vi "BuildConstructor.vi"(7 "PythonConverter_BD in":refnum<class "PyConvBD.lvclass">, 8 "error in":errorcluster, 11 "Function in":refnum<class "GrowableFunction.lvclass">) -> (0 "error out":errorcluster, 3 "Function out":refnum<class "GrowableFunction.lvclass">, 4 "constructor":string, 5 "PythonConverter_BD out":refnum<class "PyConvBD.lvclass">)   [LabVIEW 2014, in "GrowableFunction.lvclass"]
uses:
  GrowableFunction.lvclass
  Python/PythonConverter_BD/PyConvBD.lvclass
  Python/Parsing/Classes/PythonFunction/PythonFunction.lvclass/PythonFunction.ctl
  Python/Parsing/Classes/PythonFunction/PythonFunction.lvclass
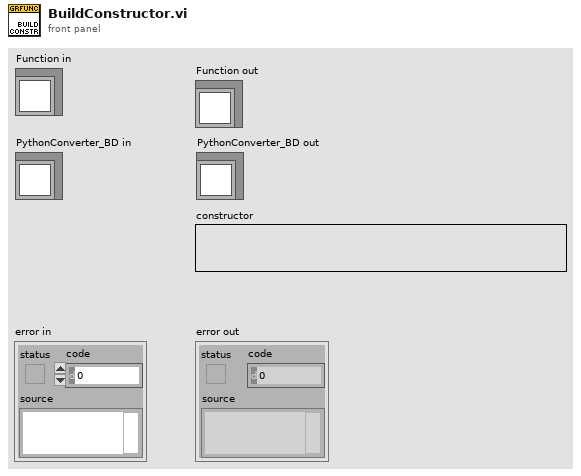
[diagram p1: front panel]
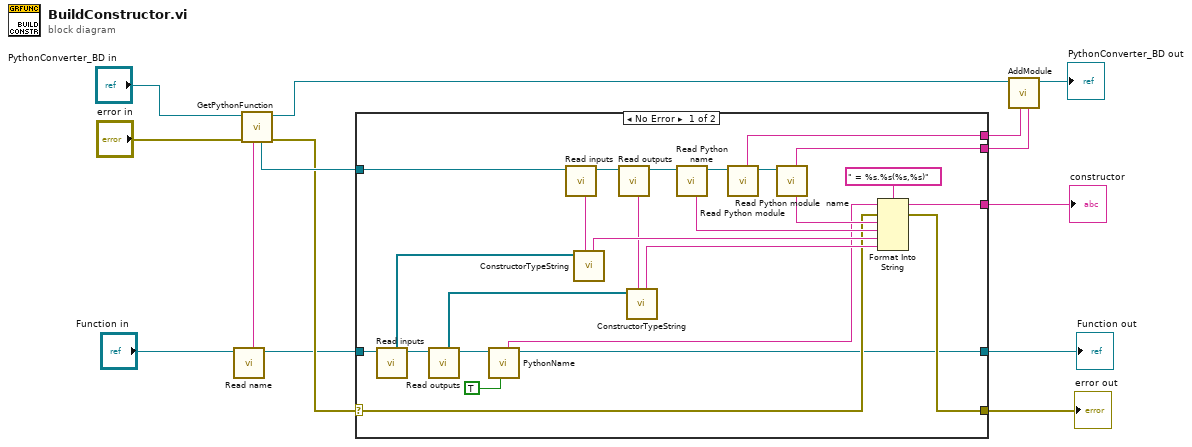
[diagram p0: block diagram]
diagram:
  n1 = call-dynamic "Read name.vi"("Node in"="Function in") -> ("Node out"=w2:refnum<class "GrowableFunction.lvclass">, "name"=w3:string)  [unwired: 7 in]
  n2 = call "GetPythonFunction.vi"("function name"=w3, "error in"="error in", "PythonConverter_BD in"="PythonConverter_BD in") -> ("error out"=w10:errorcluster, "PythonConverter_BD out"=w8:refnum<class "PyConvBD.lvclass">, "Python function"=w11:refnum<class "PythonFunction.lvclass">)  [unwired: 4 in]
  n3 = case shown="No Error" w10 {
    selector: w10 -> [w17 w40]
    tunnel: [w34 w40] -> w14
    tunnel: [w33 _] -> w13
    tunnel: w11 -> [w24 _]
    tunnel: [w32 _] -> w7
    tunnel: [w31 _] -> w6
    tunnel: w2 -> [w23 w39]
    tunnel: [w16 w39] -> w1
    frame No Error {
      n4 = call-dynamic "Read inputs.vi"("Node in"=w23) -> ("Node out"=w21:refnum<class "GrowableFunction.lvclass">, "inputs"=w22:refnum<class "Terminal.lvclass">[])  [unwired: 7 in]
      n5 = call-dynamic "Read outputs.vi"("Node in"=w21) -> ("Node out"=w19:refnum<class "GrowableFunction.lvclass">, "outputs"=w20:refnum<class "Terminal.lvclass">[])  [unwired: 7 in]
      n6 = call-dynamic "PythonName.vi"("add self"=TRUE, "Node in"=w19) -> ("Node out"=w16:refnum<class "GrowableFunction.lvclass">, "name"=w18:string)  [unwired: 6 in, 2 out]
      n7 = call "Read inputs.vi"("PythonFunction in"=w24) -> ("PythonFunction out"=w25:refnum<class "PythonFunction.lvclass">, "inputs"=w26:string)  [unwired: 7 in]
      n8 = call "ConstructorTypeString.vi"("list"=w26, "terminals"=w22) -> ("constructor string"=w37:string)  [unwired: 7 in]
      n9 = call "Read outputs.vi"("PythonFunction in"=w25) -> ("PythonFunction out"=w27:refnum<class "PythonFunction.lvclass">, "outputs"=w28:string)  [unwired: 7 in]
      n10 = call "ConstructorTypeString.vi"("list"=w28, "terminals"=w20) -> ("constructor string"=w36:string)  [unwired: 7 in]
      n11 = call "Read Python name.vi"("PythonFunction in"=w27) -> ("PythonFunction out"=w30:refnum<class "PythonFunction.lvclass">, "Python name"=w38:string)  [unwired: 7 in]
      n12 = call "Read Python module.vi"("PythonFunction in"=w30) -> ("PythonFunction out"=w29:refnum<class "PythonFunction.lvclass">, "Python module"=w32:string)  [unwired: 7 in]
      n13 = call "Read Python module  name.vi"("PythonFunction in"=w29) -> ("Python module  name"=w31:string)  [unwired: 7 in, 1 out]
      n14 = Format Into String(format string=" = %s.%s(%s,%s)", initial string=w18, error in=w17, w31, w38, w37, w36) -> (resulting string=w33:string, error out=w34:errorcluster)
    }
    frame Error {
    }
  }
  "error out" <- w14
  "Function out" <- w1
  "constructor" <- w13
  n15 = call "AddModule.vi"("python module name"=w6, "python module"=w7, "PythonConverter_BD in"=w8) -> ("PythonConverter_BD out"=→"PythonConverter_BD out":refnum<class "PyConvBD.lvclass">)  [unwired: 5 in, 1 out]
